vi "cDAQ_VI_Leo_Simplified.vi"() -> ()   [LabVIEW 2022 SP3]
uses:
  <vilib>/addons/control/pid/autopid.llb/PID autotuning parameters.ctl
  <vilib>/Analysis/baseanly.llb/Mean (DBL).vi
  <vilib>/DAQmx/read.llb/DAQmx Read (Analog 1D Wfm NChan NSamp).vi
  <vilib>/DAQmx/configure/timing.llb/DAQmx Timing (Sample Clock).vi
  STOP_GLOBAL.vi
  <vilib>/addons/control/pid/pid.llb/PID Lead-Lag (DBL).vi
  <vilib>/addons/control/pid/pid.llb/PID Gain Schedule (DBL).vi
  <vilib>/addons/control/pid/autopid.llb/PID Online Autotuning (Step Closed Loop).vi
  <vilib>/addons/control/pid/pid.llb/PID Advanced (DBL).vi
  <vilib>/addons/control/pid/pid.llb/PID (DBL).vi
  <vilib>/DAQmx/miscellaneous.llb/DAQmx Fill In Error Info.vi
  <vilib>/Analysis/NI_AALBase.lvlib
  <vilib>/addons/control/pid/NI_PID_pid.lvlib
  <vilib>/ptbypt/NI_PtbyPt.lvlib
  <vilib>/addons/control/pid/NI_PID_autopid.lvlib
  <resource>/objmgr/daqmx.rc
panel:
  out "Runtime Passed?":bool
  out "Stop":bool
  out "Elapsed Time (s)":dbl
  out "2nd Loop Time":dbl
  out "Numeric":i32
  out "Array":dbl[](array[numeric])
  in  "RunTime":dbl
  out "Entire Runtime":dbl
  out "Actual Clock Rate":dbl
  in  "MV:":dbl(slide)=30.8641975308642 scale=0.0..5.067 scale format="%.1f"
  in  "autotuning parameters":T1={"type of controller"=0, "relay cycles"=3, "relay amplitude"=1.0, "control specifications"=2, "PV noise level"=0.1} {"PV noise level" format="%.2f"; "control specifications" items=["normal", "fast", "slow"]; "relay amplitude" format="%.2f"; "type of controller" items=["P", "PI", "PID"]}
  in  "PID gain schedule":T2(array[cluster])=[{"PID gains"={"Kc"=7.0, "Ti"=0.001, "Td"=0.0}, "max value"=0.0}] {"max value" format="%.2f"; "PID gains"."Td" format="%#.3g"; "PID gains"."Ti" format="%#.3g"; "PID gains"."Kc" format="%#.3g"}
  out "error out 4":errorcluster
  out "Setpoint profile":dbl
  out "Voltage Output":dynamicdata(graph)
  out "Second Pressure Transducer":cluster{dbl[], dbl[]}(graph)
  out "Second Pressure Transducer":dynamicdata(graph)
  out "Servo Voltage Output":cluster{dbl[], dbl[]}(graph)
  in  "Tab Control":T3(tab)
  in  "Channel Array":dbl[](array[numeric]) format="%_3g"
  out "error out 5":errorcluster
  in  "stop":bool
  in  "Array 2":dbl[](array[slide]) scale=0.0..1.0
  out "Waveform Chart":cluster{"SP":dbl, dbl}(graph)
  out "Output":dbl(slide) scale=1.0..5.067
  out "Process Variable vs Setpoint":cluster{dbl[], dbl[]}[](graph)
  out "error out":errorcluster
  in  "Error":dbl
  in  "Scaling Factor":dbl
  in  "x0":dbl
  out "element":dbl
  out "MVT Process variable":dbl
  out "MVT Setpoint":dbl
  out "Gain Index":i32
  in  "SP":dbl format="%.2f"
  out "PID gains out":T4={"proportional gain (Kc)"=1.0, "integral time (Ti, min)"=0.01, "derivative time (Td, min)"=0.0} {"derivative time (Td, min)" format="%.3f"; "integral time (Ti, min)" format="%.3f"; "proportional gain (Kc)" format="%.3f"}
  in  "Insert Gain":bool
  out "output":dbl format="%.2f"
  in  "Autotune":bool
  in  "Reinitialize":bool
  in  "Automatic":bool=TRUE
  in  "Replace Gain":bool
  in  "alpha":dbl=nan format="%.2f"
  out "tuned PID gains":T4={"proportional gain (Kc)"=1.0, "integral time (Ti, min)"=0.01, "derivative time (Td, min)"=0.0} {"derivative time (Td, min)" format="%.3f"; "integral time (Ti, min)" format="%.3f"; "proportional gain (Kc)" format="%.3f"}
  out "Steps on Servo":dbl[](array[numeric])
  out "Elapsed Time (s) 2":dbl caption="Elapsed Time (s)"
  out "HAS 3 SECONDS PASSED?":bool
  in  "PRESS TO START":bool
  out "All Channel Graph":cluster{dbl[], dbl[]}[](graph)
  out "Thrust":cluster{dbl[], dbl[]}(graph)
  out "Chamber Pressure":cluster{dbl[], dbl[]}(graph)
  out "Supply Pressure":cluster{dbl[], dbl[]}(graph)
  out "MassFlow":cluster{dbl[], dbl[]}(graph)
  out "Temperature":cluster{dbl[], dbl[]}(graph)
  out "error out 3":errorcluster caption="error out"
  out "error out 2":errorcluster
  in  "rate":dbl=1000.0 format="%0.2f"
  in  "number of samples":i32=100
  in  "File Format":string
  in  "File Name Out":string
  in  "Data Collection Folder":path
  out "Temperature":dynamicdata(graph)
  out "Numeric 2":i32
  out "Thrust lb":dynamicdata(graph)
  in  "Types of Testing":enum32{"Test Firing", "Cold Flow Rig"}(tab)
  out "Saving Data":bool
  out "Filename Out":path
  in  "Collect Data?":bool=TRUE caption="Enable"
  in  "Collect Data? 2":bool=TRUE caption="Enable"
  out "Saving Data":bool
  out "Filename Out":path
  out "Supply Pressure PSI":dynamicdata(graph)
  out "Mass Flow L/min":dynamicdata(graph)
  out "Chamber Pressure":dynamicdata(graph)
  # "Control Loop"
  # "DATA LOGGING INFORMATION"
  # "ANALOG VOLTAGE OUTPUT"
  # "RESULTS"
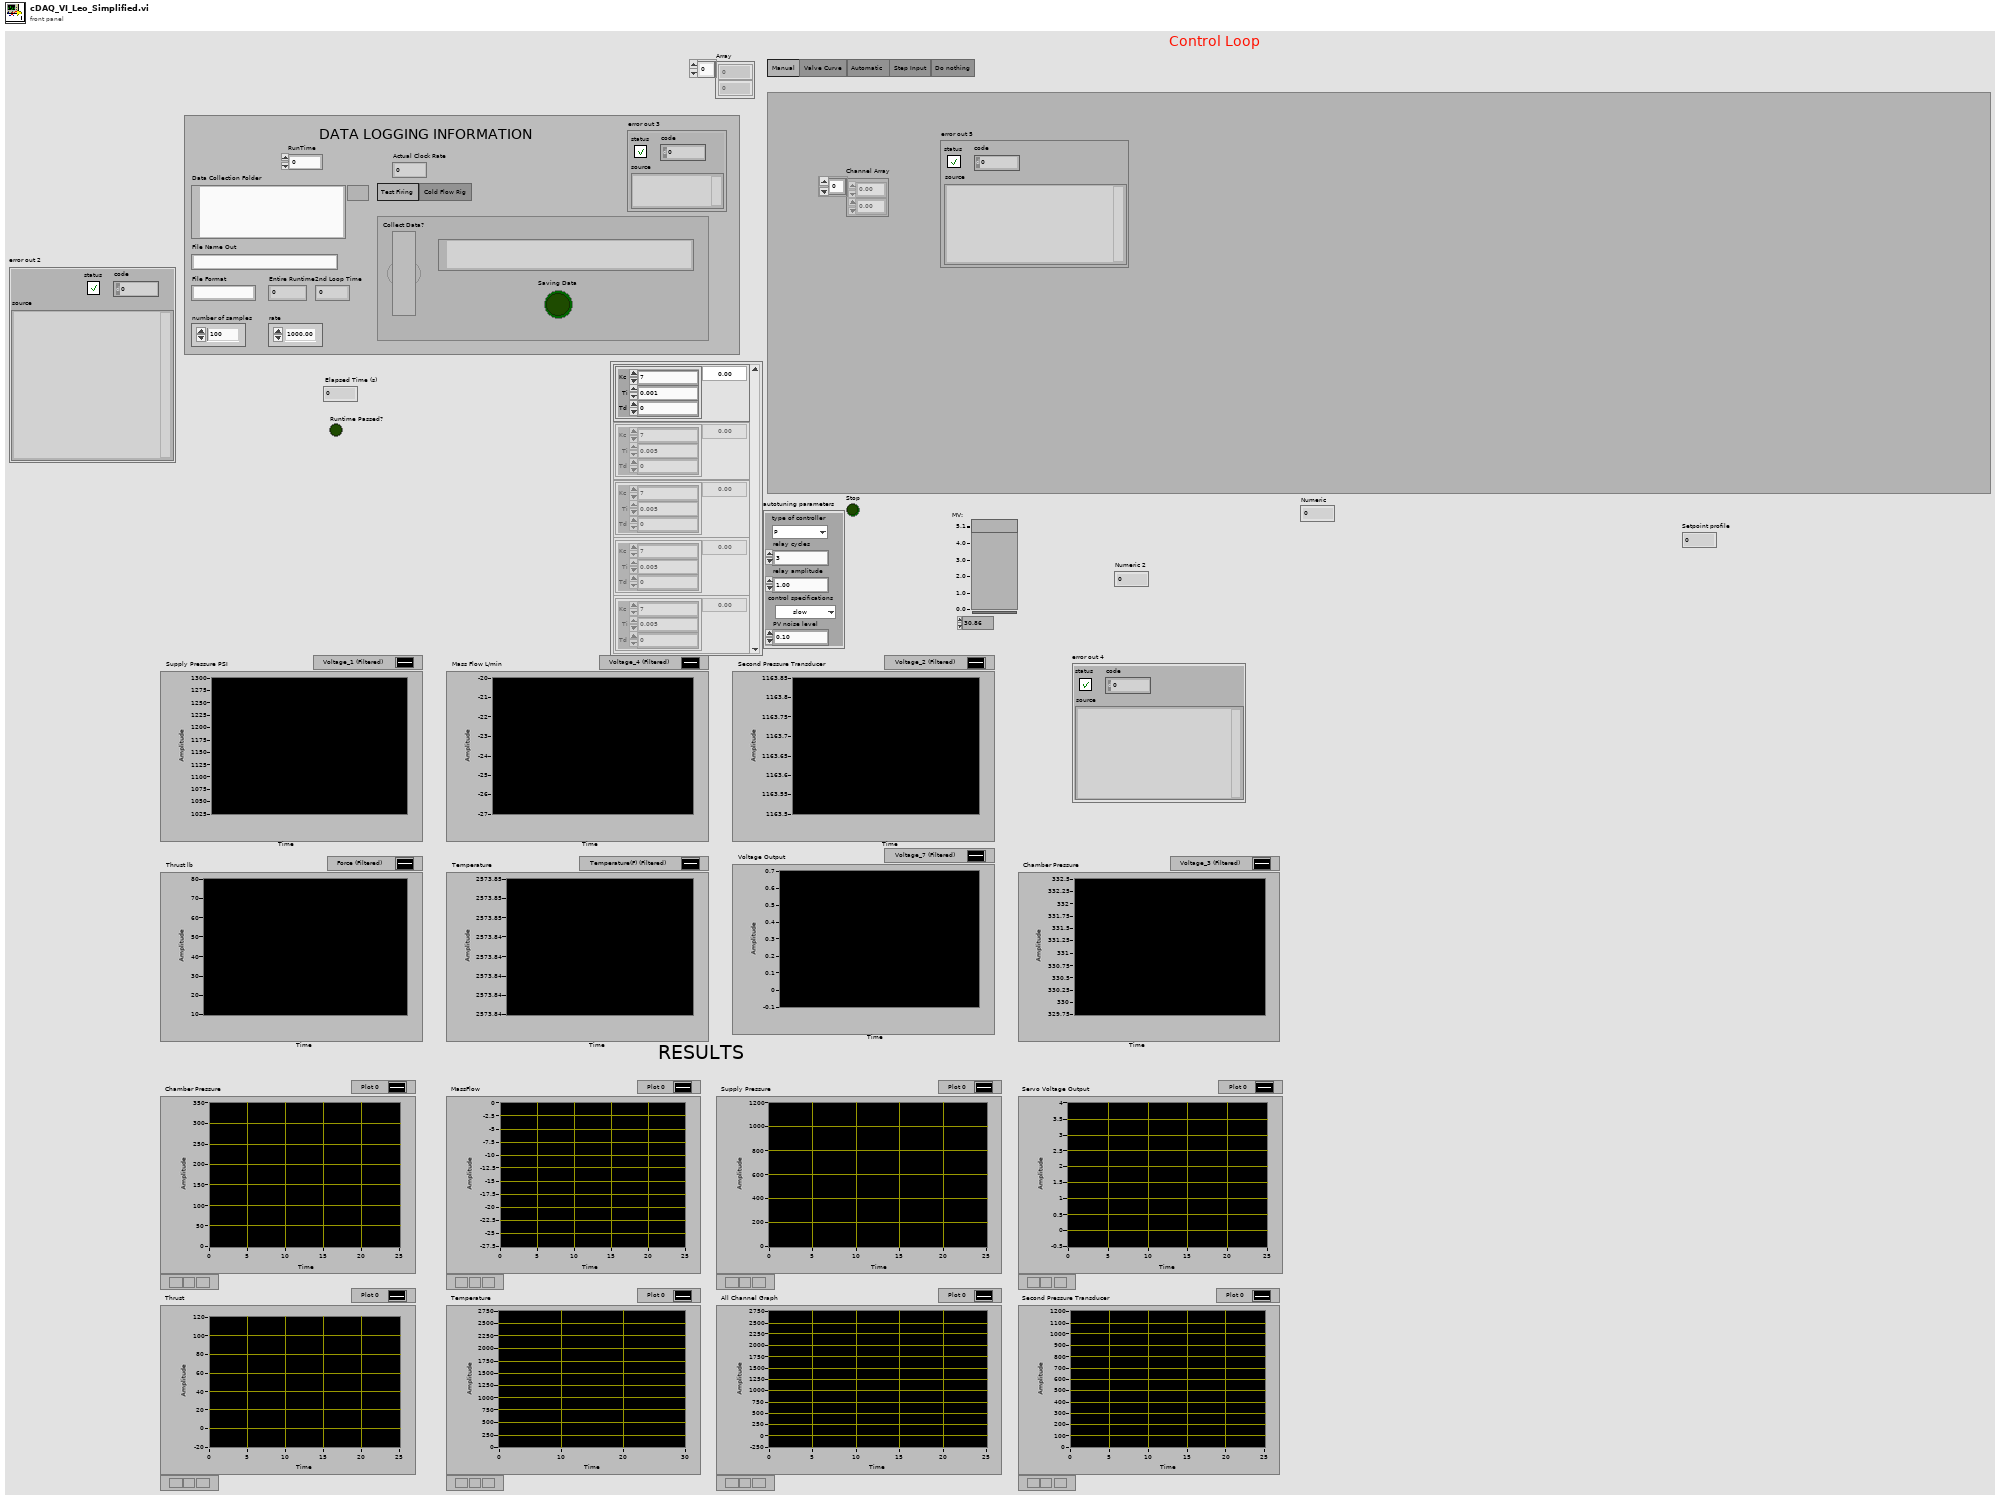
[diagram p1: front panel]
types:
  T1 = typedef "PID autotuning parameters.ctl" = cluster{"type of controller":u16, "relay cycles":i32, "relay amplitude":dbl, "control specifications":u16, "PV noise level":dbl}
  T2 = cluster{"PID gains":cluster{"Kc":dbl, "Ti":dbl, "Td":dbl}, "max value":dbl}[]
  T3 = enum32{"Manual", "Valve Curve", "Automatic", "Step Input", "Do nothing"}
  T4 = cluster{"proportional gain (Kc)":dbl, "integral time (Ti, min)":dbl, "derivative time (Td, min)":dbl}
  T5 = cluster{"tuned PID gains":cluster{"proportional gain (Kc)":dbl, "integral time (Ti, min)":dbl, "derivative time (Td, min)":dbl}, "SP":dbl}
  T6 = cluster{"PID gains":cluster{"Kc":dbl, "Ti":dbl, "Td":dbl}, "max value":dbl}
  T7 = cluster{"tuned PID gains":cluster{"proportional gain (Kc)":dbl, "integral time (Ti, min)":dbl, "derivative time (Td, min)":dbl}, "max value":dbl}
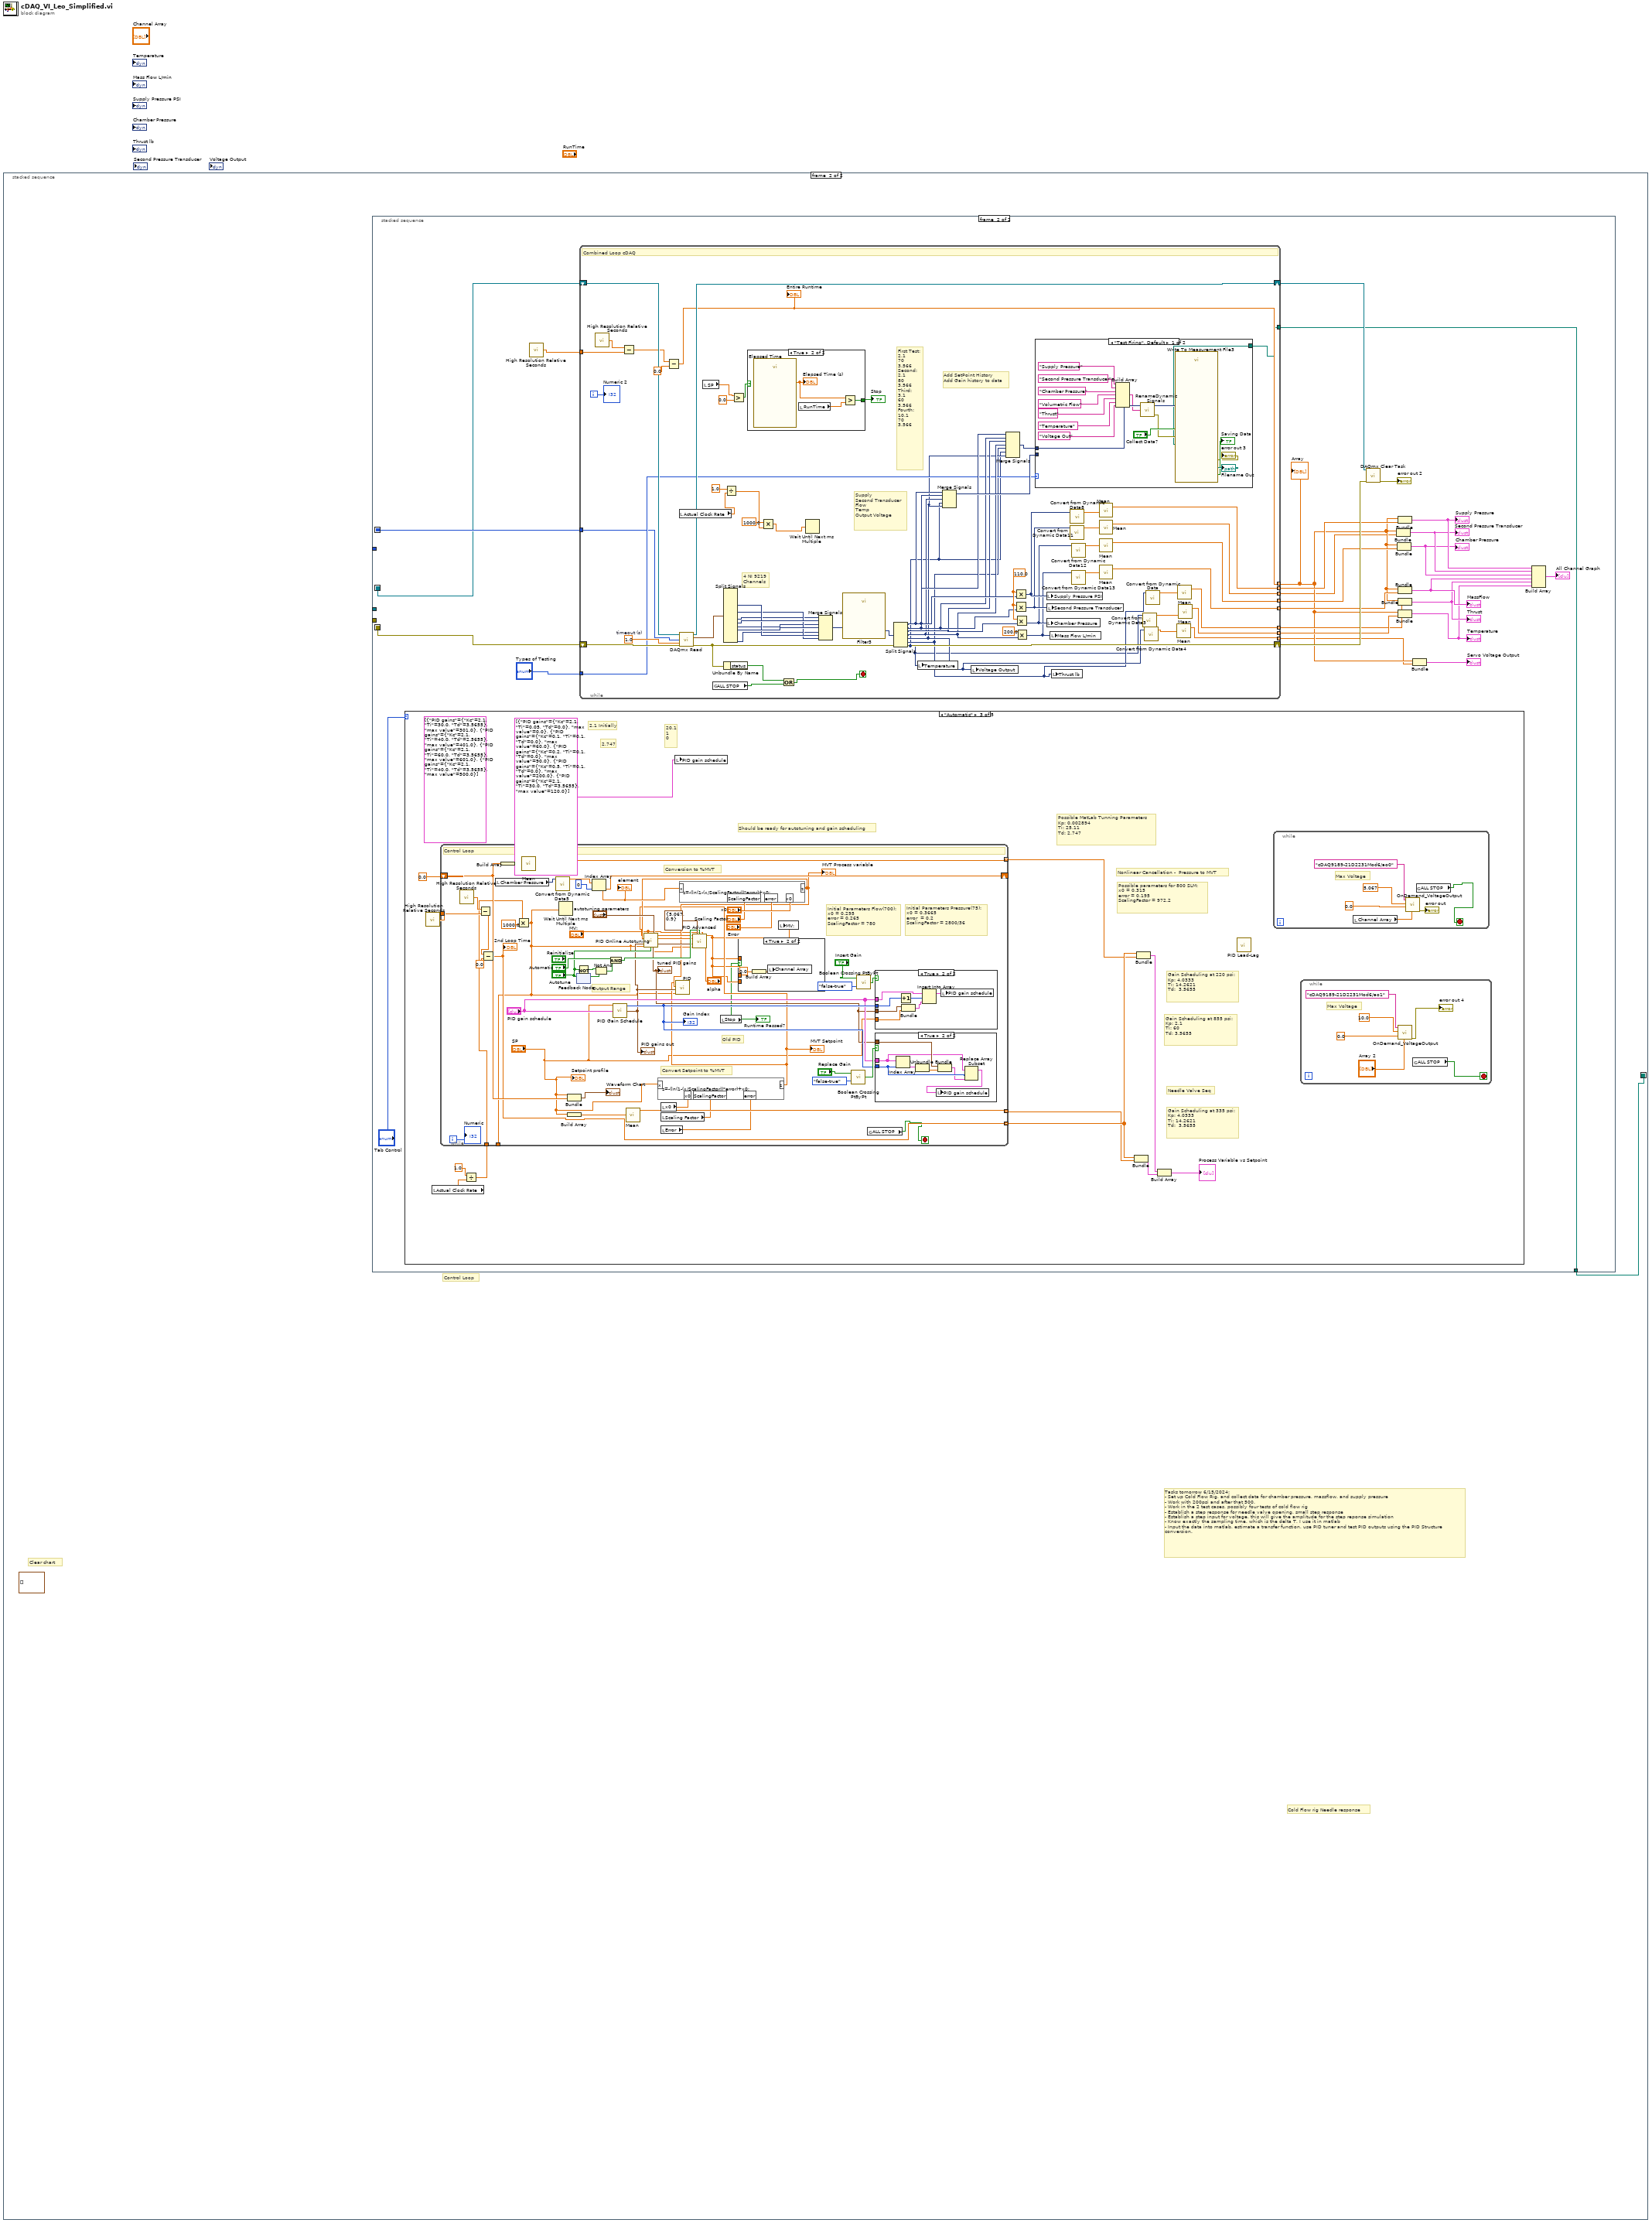
[diagram p0: block diagram]
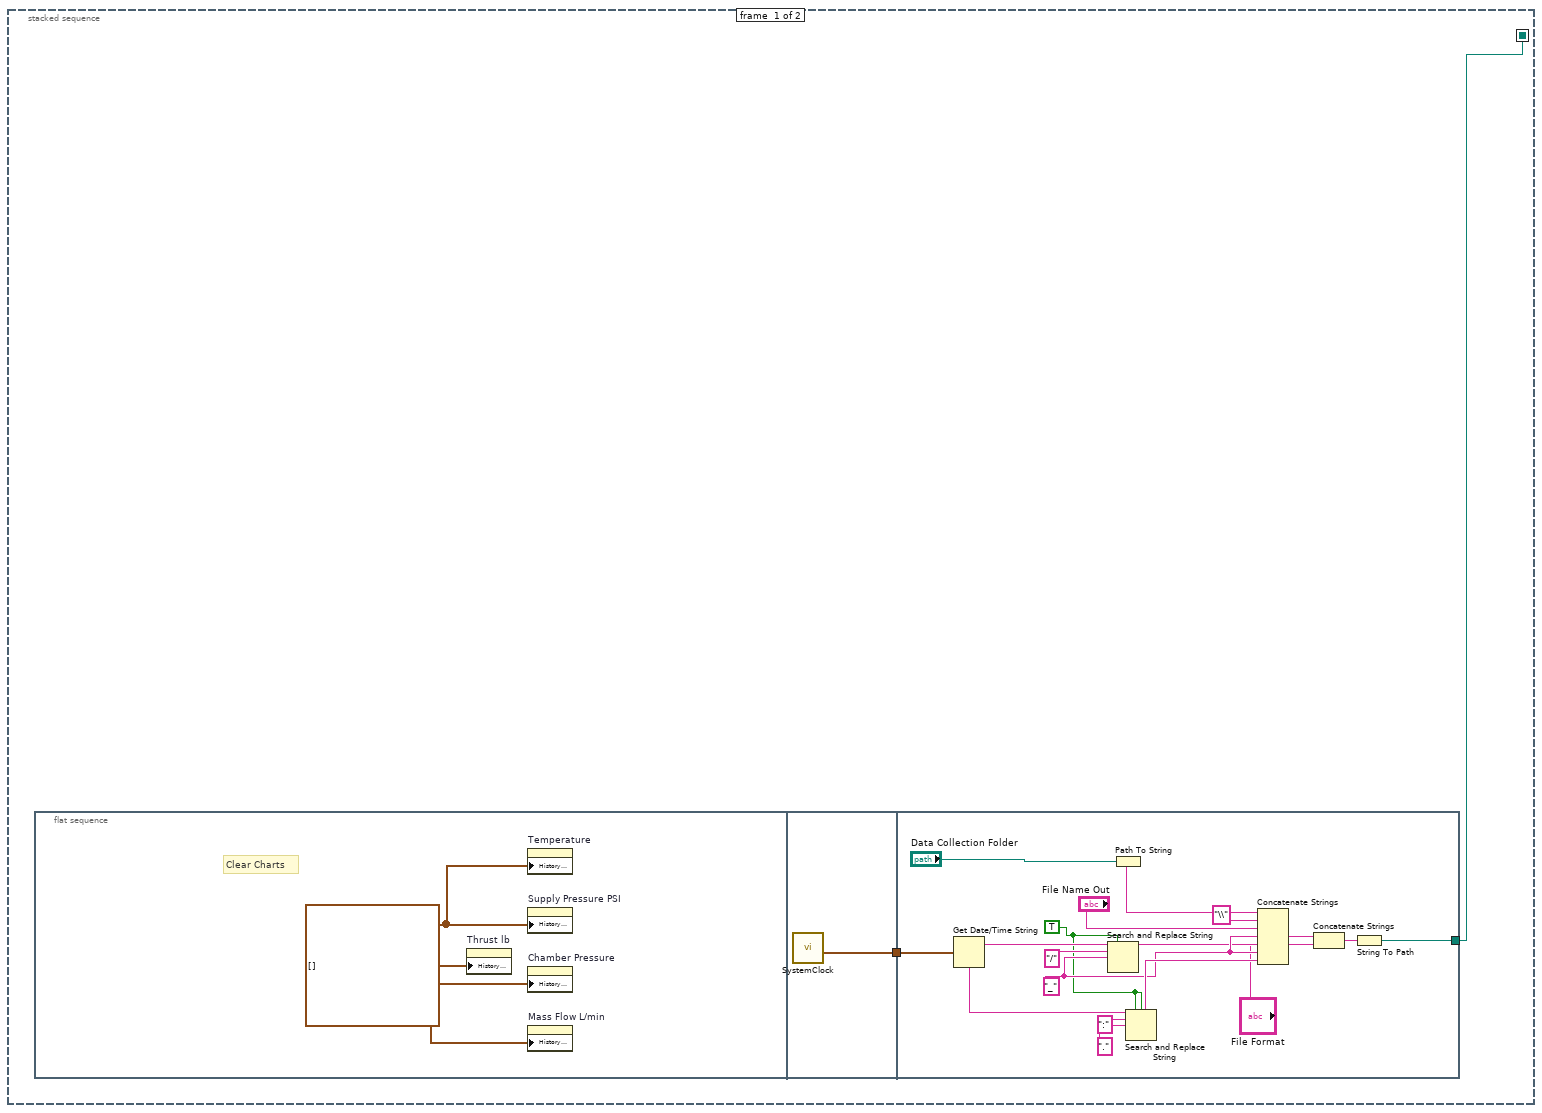
[diagram p2: hidden frame]
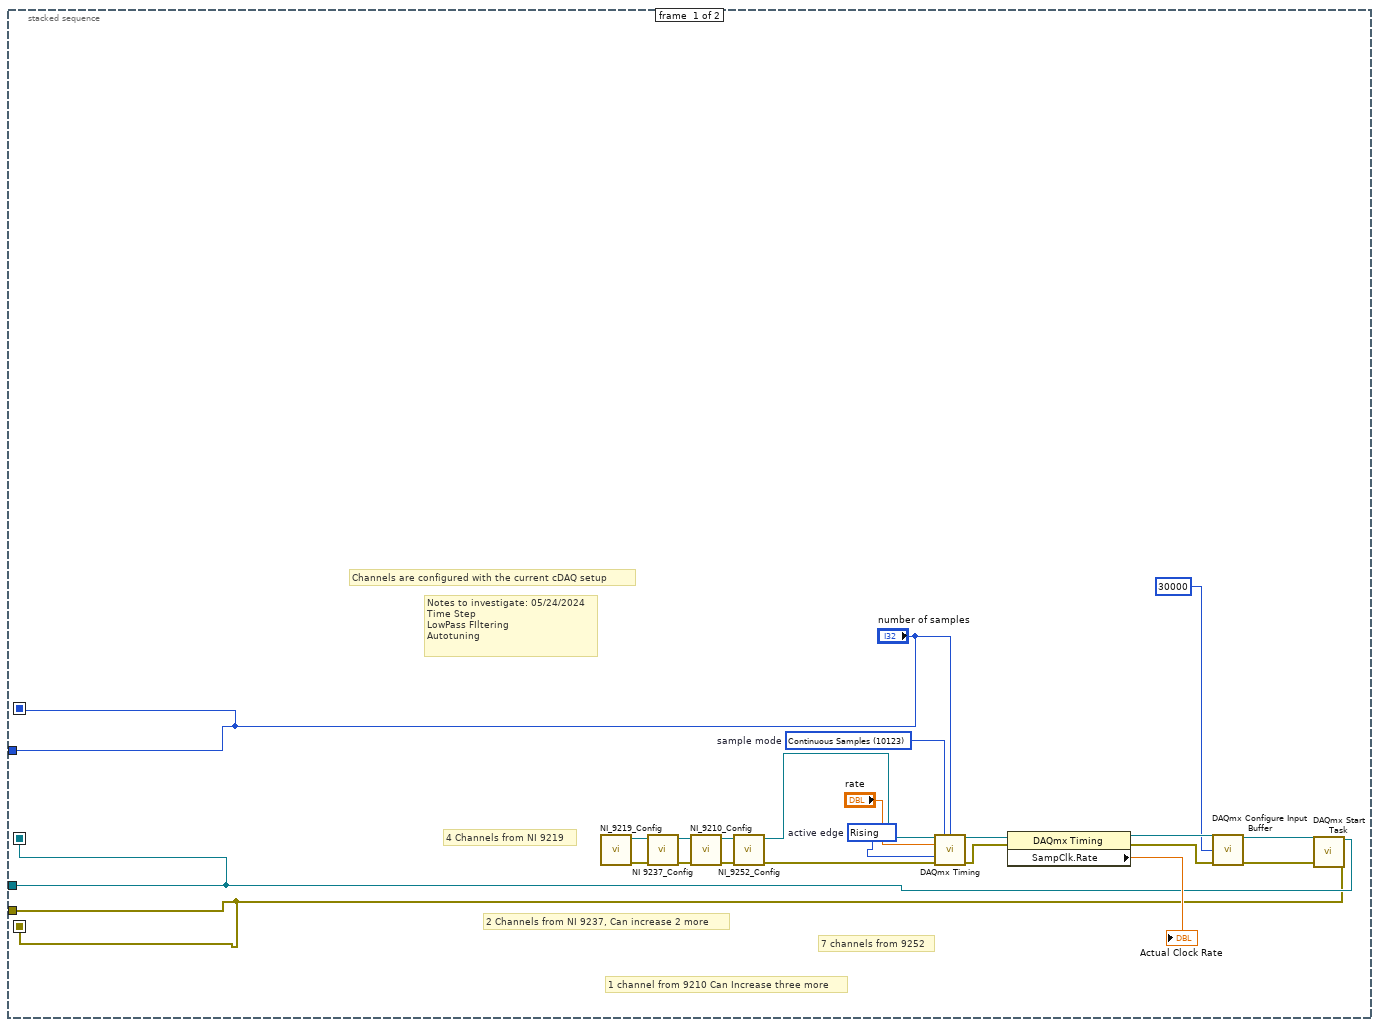
[diagram p3: hidden frame]
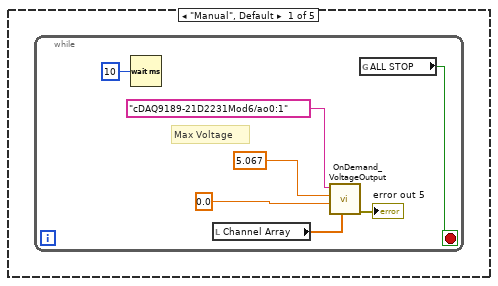
[diagram p4: hidden frame]
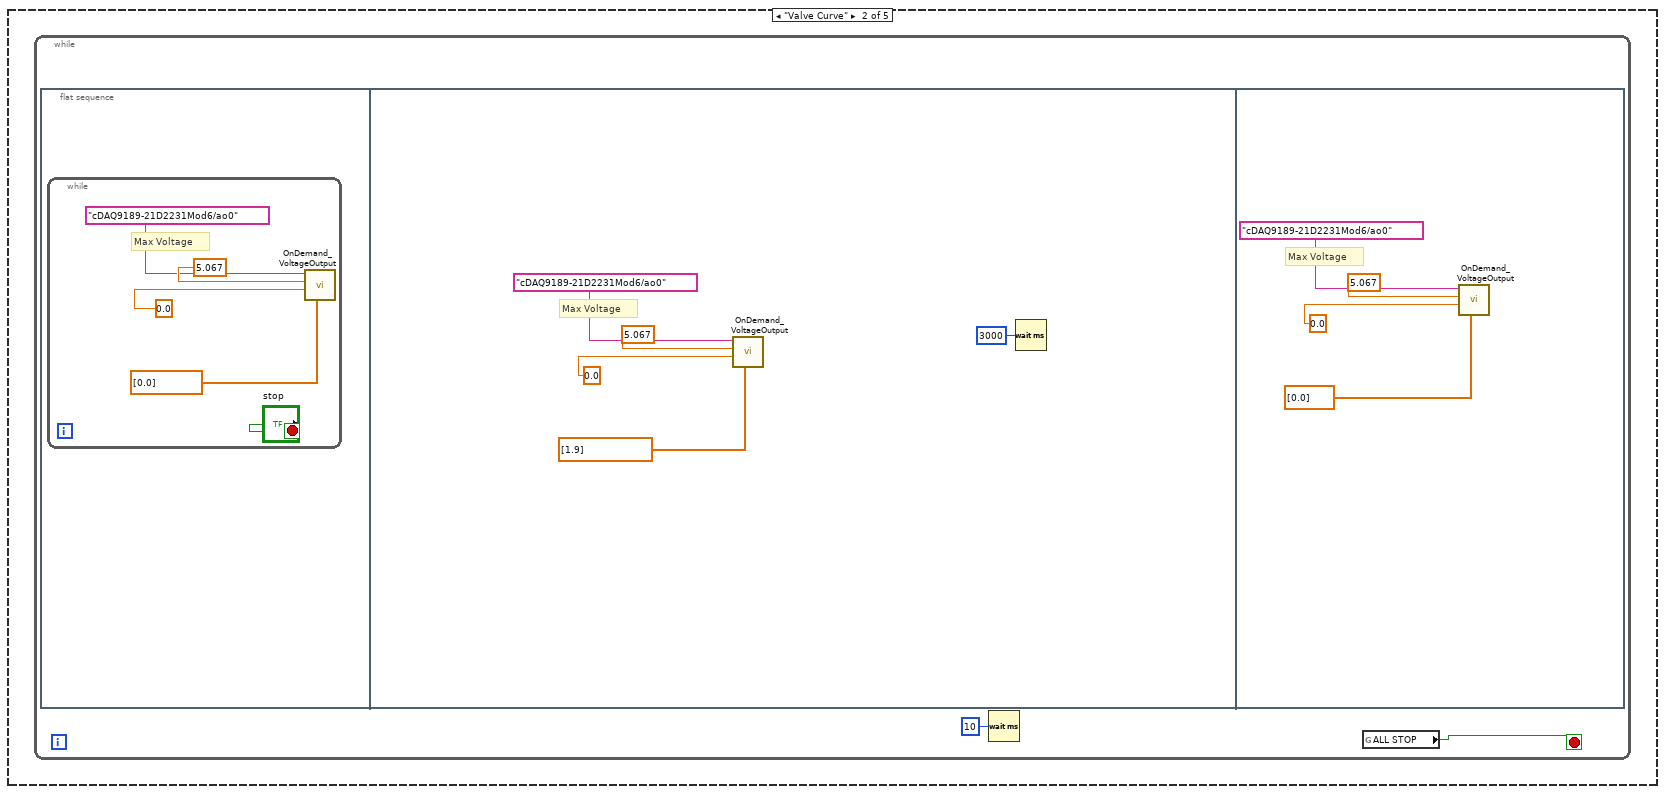
[diagram p5: hidden frame]
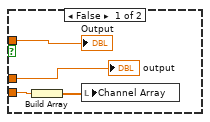
[diagram p6: hidden frame]
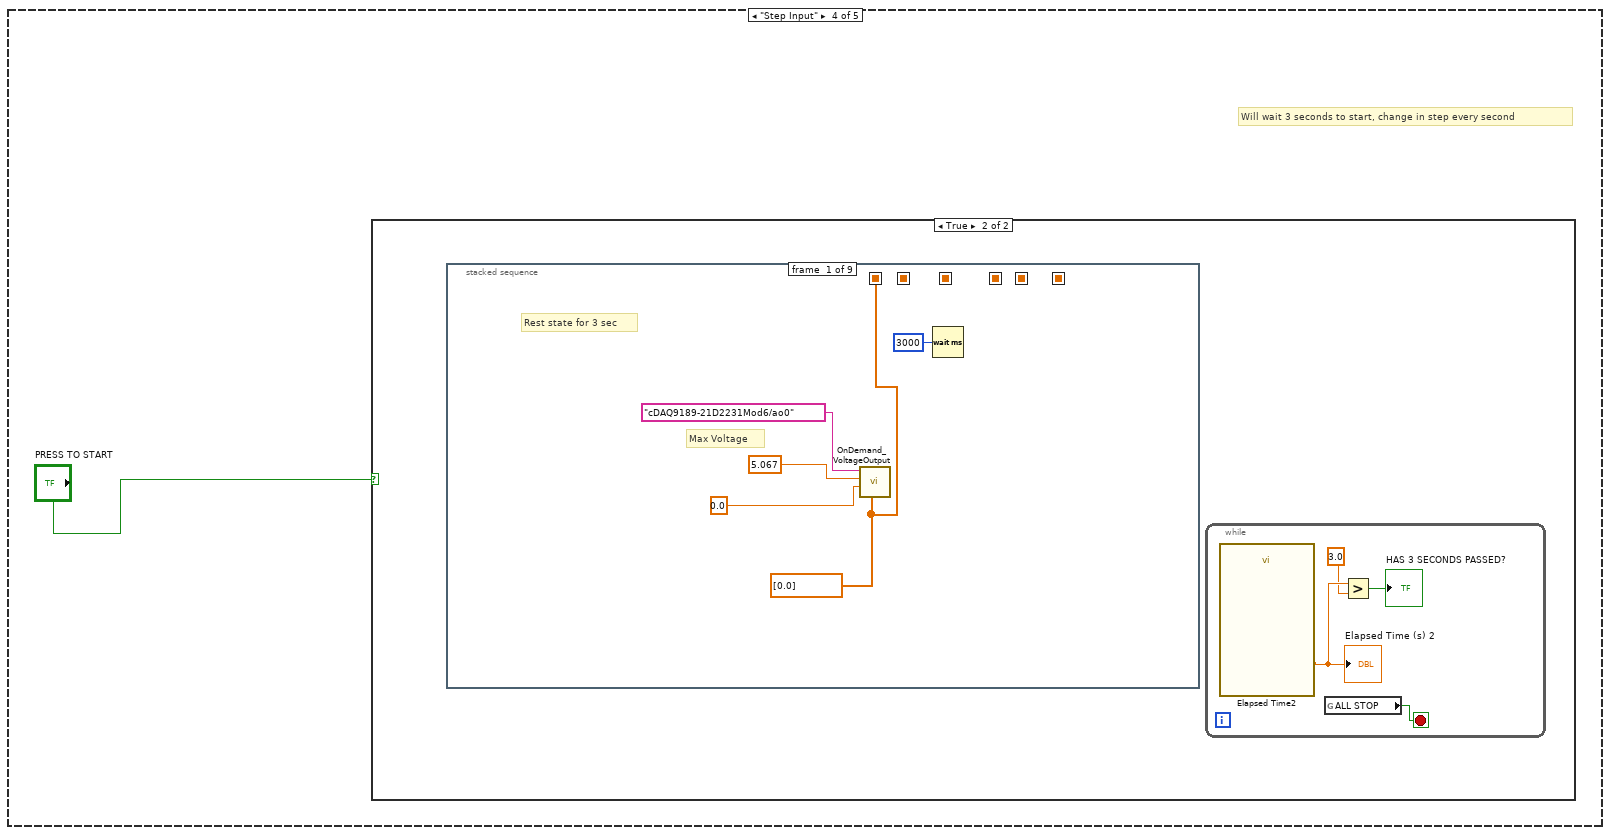
[diagram p9: hidden frame]
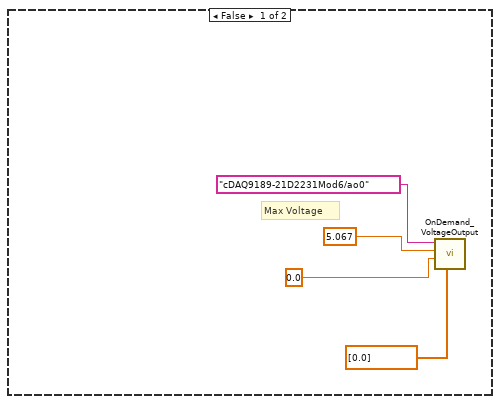
[diagram p10: hidden frame]
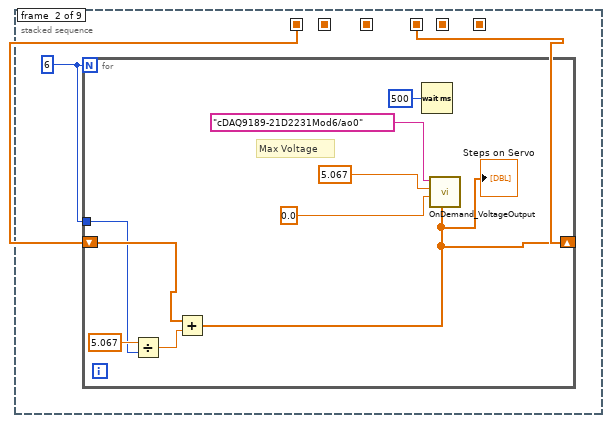
[diagram p11: hidden frame]
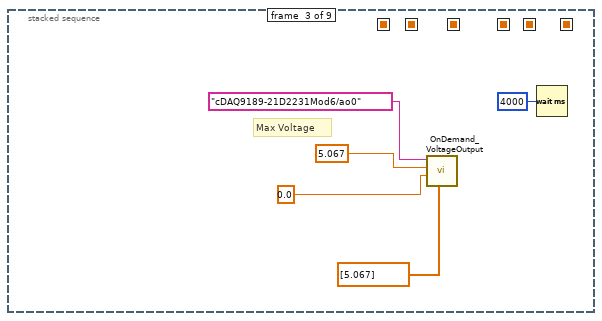
[diagram p12: hidden frame]
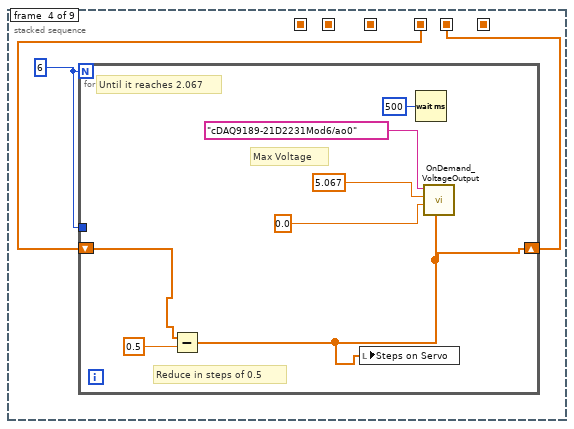
[diagram p13: hidden frame]
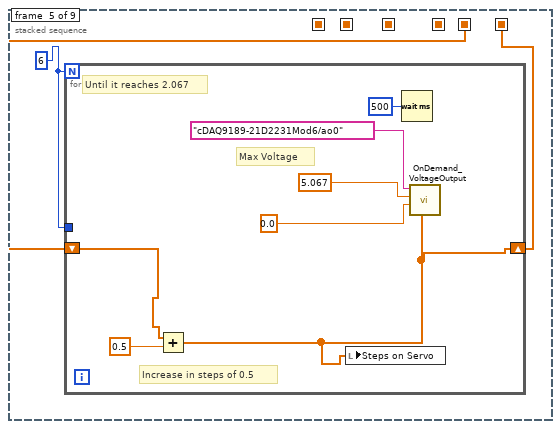
[diagram p14: hidden frame]
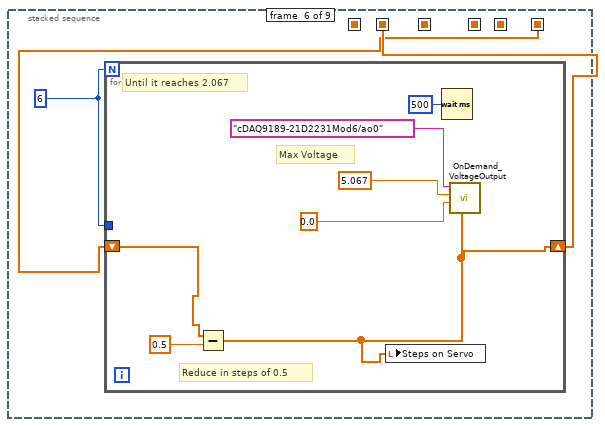
[diagram p15: hidden frame]
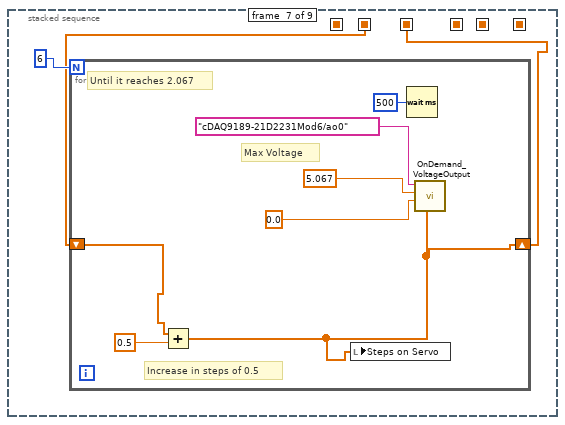
[diagram p16: hidden frame]
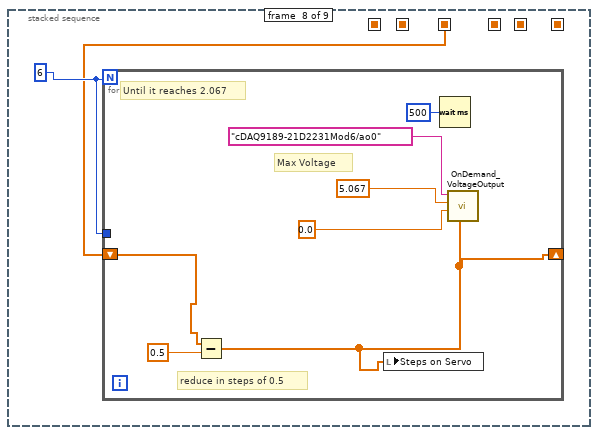
[diagram p17: hidden frame]
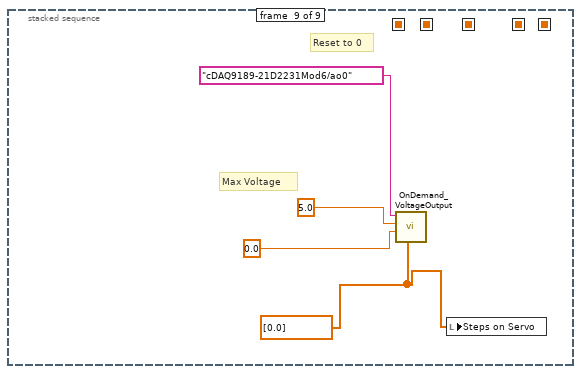
[diagram p18: hidden frame]
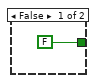
[diagram p20: hidden frame]
diagram:
  n1 = stacked-sequence {
    seq-local: [w1 _] -> [_ w23]
    frame #0 {
      n2 = flat-sequence {
        tunnel: [w4] -> w2
        tunnel: w2 -> [w11]
        tunnel: [w10] -> w1
        frame #0 {
          w3 = waveform(dbl)[] []
          # "Clear Charts"
          n3 = property on="Thrust lb" class="WFChart (strict)"("History Data"=w3) -> ()  [unwired: 2 in, 2 out]
          n4 = property on="Temperature" class="WFChart (strict)"("History Data"=w3) -> ()  [unwired: 2 in, 2 out]
          n5 = property on="Supply Pressure PSI" class="WFChart (strict)"("History Data"=w3) -> ()  [unwired: 2 in, 2 out]
          n6 = property on="Chamber Pressure" class="WFChart (strict)"("History Data"=w3) -> ()  [unwired: 2 in, 2 out]
          n7 = property on="Mass Flow L/min" class="WFChart (strict)"("History Data"=w3) -> ()  [unwired: 2 in, 2 out]
        }
        frame #1 {
          n8 = call "SystemClock.vi"() -> ("LabVIEW Time Stamp"=w4:timestamp)  [unwired: 9 in, 2 out]
        }
        frame #2 {
          w6 = TRUE ("replace all? (F)")
          w19 = "_" ("string")
          n9 = Get Date/Time String(seconds (now)=w11) -> (date string=w13:string, time string=w16:string)  [unwired: 2 in]
          n10 = Search and Replace String(replace all?=w6, input string=w13, search string="/", replace string=w19) -> (result string=w15:string)  [unwired: 4 in, 3 out]
          n11 = Path To String(path="Data Collection Folder") -> (string=w8:string)
          n12 = Search and Replace String(replace all?=w6, case sensitive?=w6, input string=w16, search string=":", replace string="." ("replace string (\"\")")) -> (result string=w20:string)  [unwired: 3 in, 3 out]
          n13 = Concatenate Strings(w8, "\\" ("string"), "File Name Out", w19, w15, w19, w20) -> (w21:string)
          n14 = Concatenate Strings(w21, "File Format") -> (w22:string)
          n15 = String To Path(string=w22) -> (path=w10:path)
        }
      }
    }
    frame #1 {
      (unwired) cluster{"setpoint":dbl, dbl}[] [] ("History Data")
      # "Cold Flow rig Needle response"
      # "Tasks tomorrow 6/15/2024:\n- Set up Cold Flow Rig, and collect data for chamber pressure, massflow, and supply pressure\n- Work with 200psi and after that 500.\n- Work in the 2 test cases, possibly four tests of cold flow rig\n- Establish a step response for needle valve opening, small step response\n- Establish a step input for voltage, this will give the amplitude for the step reponse simulation\n- Know exactly the sampling time, which is the delta T, I use it in matlab\n- Input the data into matlab, estimate a transfer function, use PID tuner and test PID outputs using the PID Structure\nconversion."
      # "Control Loop"
      # "Clear chart"
      n16 = stacked-sequence {
        seq-local: ["number of samples" _] -> [_ w50]
        seq-local: [w25 _] -> [_ w49]
        seq-local: [w24 _] -> [_ w48]
        tunnel: w23 -> [_ w46]
        tunnel: [w25 _] -> _
        tunnel: [w24 _] -> _
        tunnel: ["number of samples" _] -> _
        frame #0 {
          w28 = 10123 items=["Finite Samples"=10178, "Continuous Samples"=10123, "Hardware Timed Single Point"=12522]  # sample mode
          w27 = 10280 items=["Rising"=10280, "Falling"=10171]  # active edge
          # "Notes to investigate: 05/24/2024\nTime Step\nLowPass FIltering\nAutotuning"
          # "Channels are configured with the current cDAQ setup"
          # "7 channels from 9252"
          # "1 channel from 9210 Can Increase three more"
          # "2 Channels from NI 9237, Can increase 2 more"
          # "4 Channels from NI 9219"
          n17 = call "NI_9219_Config.vi"() -> ("error out"=w38:errorcluster, "task out"=w30:refnum<k21>)  [unwired: 10 in]
          n18 = call "NI 9237_Config.vi"("error in"=w38, "task in"=w30) -> ("error out"=w32:errorcluster, "task out"=w31:refnum<k21>)  [unwired: 8 in]
          n19 = call "NI_9210_Config.vi"("error in"=w32, "task in"=w31) -> ("error out"=w34:errorcluster, "task out"=w33:refnum<k21>)  [unwired: 8 in]
          n20 = call "NI_9252_Config.vi"("error in"=w34, "task in"=w33) -> ("error out"=w36:errorcluster, "task out"=w35:refnum<k21>)  [unwired: 8 in]
          n21 = call-poly <vilib>:"DAQmx Timing.vi"("task/channels in"=w35, "sample mode"=w28, "samples per channel"="number of samples", "rate"="rate", "active edge"=w27, "error in"=w36) -> ("task out"=w39:refnum<k21>, "error out"=w40:errorcluster)  [unwired: 8 in]
          n22 = property class="DAQmx Timing"(reference=w39, error in=w40) -> (reference out=w41:refnum<k21>, error out=w42:errorcluster, "SampClk.Rate"=→"Actual Clock Rate":dbl)
          n23 = call <vilib>:"DAQmx Configure Input Buffer.vi"("task/channels in"=w41, "buffer size (in samples per channel)"=u32 30000, "error in"=w42) -> ("task out"=w44:refnum<k21>, "error out"=w43:errorcluster)  [unwired: 11 in]
          n24 = call <vilib>:"DAQmx Start Task.vi"("task/channels in"=w44, "error in"=w43) -> ("task out"=w25:refnum<k21>, "error out"=w24:errorcluster)  [unwired: 12 in]
        }
        frame #1 {
          n25 = case shown="\"Automatic\"" "Tab Control" {
            frame "Manual", Default {
              n26 = while {
                stop <- w78 stop-if-true
                # "Max Voltage"
                n27 = Wait (ms)(milliseconds to wait=u32 10) -> ()  [unwired: 1 out]
                n28 = local read "Channel Array"() -> (w74:dbl[])
                n29 = call "OnDemand_VoltageOutput.vi"("Channel Array"=w74, "minimum voltage"=0.0, "maximum voltage"=5.067, "physical channels"="cDAQ9189-21D2231Mod6/ao0:1") -> ("error out"=→"error out 5":errorcluster)  [unwired: 7 in]
                n30 = global read "STOP_GLOBAL.vi" "ALL STOP"() -> (w78:bool)
              }
            }
            frame "Valve Curve" {
              n31 = while {
                stop <- w79 stop-if-true
                n32 = flat-sequence {
                  frame #0 {
                    n33 = while {
                      stop <- "stop" stop-if-true
                      # "Max Voltage"
                      n34 = call "OnDemand_VoltageOutput.vi"("Channel Array"=dbl[] [0.0], "minimum voltage"=0.0, "maximum voltage"=5.067, "physical channels"="cDAQ9189-21D2231Mod6/ao0") -> ()  [unwired: 7 in, 1 out]
                    }
                  }
                  frame #1 {
                    # "Max Voltage"
                    n35 = call "OnDemand_VoltageOutput.vi"("Channel Array"=dbl[] [1.9], "minimum voltage"=0.0, "maximum voltage"=5.067, "physical channels"="cDAQ9189-21D2231Mod6/ao0") -> ()  [unwired: 7 in, 1 out]
                    n36 = Wait (ms)(milliseconds to wait=u32 3000) -> ()  [unwired: 1 out]
                  }
                  frame #2 {
                    # "Max Voltage"
                    n37 = call "OnDemand_VoltageOutput.vi"("Channel Array"=dbl[] [0.0], "minimum voltage"=0.0, "maximum voltage"=5.067, "physical channels"="cDAQ9189-21D2231Mod6/ao0") -> ()  [unwired: 7 in, 1 out]
                  }
                }
                n38 = Wait (ms)(milliseconds to wait=u32 10) -> ()  [unwired: 1 out]
                n39 = global read "STOP_GLOBAL.vi" "ALL STOP"() -> (w79:bool)
              }
            }
            frame "Automatic" {
              (unwired) T2 [{"PID gains"={"Kc"=2.1, "Ti"=30.0, "Td"=3.5655}, "max value"=301.0}, {"PID gains"={"Kc"=2.1, "Ti"=40.0, "Td"=2.5655}, "max value"=401.0}, {"PID gains"={"Kc"=2.1, "Ti"=60.0, "Td"=3.5655}, "max value"=601.0}, {"PID gains"={"Kc"=2.1, "Ti"=40.0, "Td"=3.5655}, "max value"=500.0}] ("PID gain schedule 2")
              # "2.1 Initially"
              # "20.1\n1\n0"
              # "2.747"
              # "Should be ready for autotuning and gain scheduling"
              # "Possible parameters for 800 SLM:\nx0 = 0.315\nerror = 0.195\nScalingFactor = 972.2"
              # "Nonlinear Cancellation -  Pressure to MVT"
              # "Possible MatLab Tunning Parameters\nKp: 0.002894\nTi: 25.11\nTd: 2.747"
              # "Gain Scheduling at 335 psi:\nKp: 4.0333\nTi: 14.2621\nTd:  3.5655"
              # "Gain Scheduling at 855 psi:\nKp: 2.1\nTi: 60\nTd: 3.5655"
              # "Gain Scheduling at 220 psi:\nKp: 4.0333\nTi: 14.2621\nTd:  3.5655"
              # "Needle Valve Seq"
              n40 = call <vilib>:"High Resolution Relative Seconds.vi"() -> ("relative seconds"=w98:dbl)
              n41 = local read "Actual Clock Rate"() -> (w97:dbl)
              n42 = Divide(x=1.0, y=w97) -> (x/y=w95:dbl)
              n43 = while {
                shift-right: [w136] -> _
                shift-left: 0.0 -> [w171]
                tunnel: [w127] -> w104 mode=indexing
                tunnel: [w170] -> w102 mode=indexing
                tunnel: [w168] -> w103 mode=indexing
                tunnel: w98 -> [w131]
                tunnel: [w126] -> _
                tunnel: w95 -> [w125]
                i -> [w132]
                stop <- w120 stop-if-true
                # "Old PID"
                # "Initial Parameters Pressure(75):\nx0 = 0.3665\nerror  = 0.2\nScalingFactor = 2800/36"
                # "Initial Parameters Flow(700):\nx0 = 0.295\nerror = 0.265\nScalingFactor = 780"
                # "Convert Setpoint to %MVT"
                # "Conversion to %MVT"
                # "Output Range"
                # "Control Loop"
                n44 = call <vilib>:"High Resolution Relative Seconds.vi"() -> ("relative seconds"=w130:dbl)
                n45 = Subtract(x=w130, y=w131) -> (x-y=w129:dbl)
                n46 = Subtract(x=w129, y=0.0) -> (x-y=w127:dbl)
                "2nd Loop Time" <- w127
                n47 = local read "Chamber Pressure"() -> (w122:dynamicdata)
                n48 = Build Array(w171) -> (w169:dbl[])
                n49 = Multiply(x=w125, y=1000.0) -> (x*y=w126:dbl)
                n50 = call-poly <vilib>:"Mean.vi"("X"=w169) -> ("mean"=w170:dbl)  [unwired: 1 out]
                n51 = call "Convert from Dynamic Data5"("Dynamic Data Type"=w122) -> ("Array"=w160:dbl[])  [unwired: 3 in]
                n52 = Wait Until Next ms Multiple(millisecond multiple=w126) -> ()  [unwired: 1 out]
                n53 = Bundle("SP"="SP", w171) -> (→"Waveform Chart":cluster{"SP":dbl, dbl})  [unwired: 1 in]
                n54 = Build Array("SP") -> (w166:dbl[])
                n55 = feedback #1() -> (w155:bool)  [unwired: 1 in]
                n56 = feedback-in #1("Autotune") -> ()
                n57 = Not(x="Autotune") -> (.not. x?=w154:bool)
                n58 = Index Array(array=w160, index=0) -> (element=w136:dbl)
                "element" <- w136
                n59 = Not And(1:w155, 2:w154) -> (0:w153:bool)
                n60 = And(x="Automatic", y=w153) -> (x .and. y?=w149:bool)
                n61 = call-poly <vilib>:"PID Gain Schedule.vi"("PID gain schedule"="PID gain schedule", "gain scheduling value"="SP") -> ("PID gains out"=w139:T4, "index out"=w141:i32)  [unwired: 2 in]
                "Gain Index" <- w141
                "PID gains out" <- w139
                n62 = call-poly <vilib>:"Mean.vi"("X"=w166) -> ("mean"=w168:dbl)  [unwired: 1 out]
                n63 = local read "x0"() -> (w165:dbl)
                n64 = local read "Scaling Factor"() -> (w156:dbl)
                n65 = local read "Error"() -> (w164:dbl)
                n66 = formula code="z=-(ln(1-(x/ScalingFactor))*error)+x0;"("x"="SP", "x0"=w165, "ScalingFactor"=w156, "error"=w164) -> ("z"=w134:dbl)
                "MVT Setpoint" <- w134
                n67 = formula code="z=-(ln(1-(x/ScalingFactor))*error)+x0;"("x"=w136, "x0"="x0", "ScalingFactor"="Scaling Factor", "error"="Error") -> ("z"=w135:dbl)
                "MVT Process variable" <- w135
                n68 = call-poly <vilib>:"PID Online Autotuning.vi"("setpoint"=w134, "manipulated variable"="MV:", "autotuning parameters"="autotuning parameters", "process variable"=w135, "PID gains in"=w139, "dt (s)"=w126, "autotune? (F)"="Autotune") -> ("setpoint out"=w148:dbl, "process variable out"=w147:dbl, "PID gains out"=w146:T4, "tuned PID gains"=w137:T4)  [unwired: 4 in, 1 out]
                "tuned PID gains" <- w137
                n69 = call-poly <vilib>:"PID.vi"("dt (s)"=w126, "PID gains"=w139, "process variable"=w135, "setpoint"=w134) -> ()  [unwired: 6 in, 2 out]
                n70 = call-poly <vilib>:"PID Advanced.vi"("setpoint"=w148, "output range"=cluster{"output high":dbl, "output low":dbl} {"output high"=5.067, "output low"=0.9}, "auto? (T)"=w149, "manual control"="MV:", "process variable"=w147, "alpha"="alpha", "PID gains"=w146, "dt (s)"=w126) -> ("output"=w123:dbl)  [unwired: 6 in, 1 out]
                n71 = local read "Stop"() -> (w119:bool)
                "Runtime Passed?" <- w119
                n72 = case shown="True" w119 {
                  tunnel: w123 -> [w176 _]
                  tunnel: w123 -> [w175 _]
                  tunnel: w123 -> [w173 _]
                  frame False {
                    n73 = Build Array(w173) -> (w174:dbl[])
                    n74 = local write "Channel Array"(w174) -> ()
                    "Output" <- w176
                    "output" <- w175
                  }
                  frame True {
                    n75 = Build Array(0.0 ("element")) -> (w178:dbl[])
                    n76 = local write "Channel Array"(w178) -> ()
                  }
                }
                n77 = local write "MV:"(w123) -> ()
                n78 = call <vilib>:"Boolean Crossing PtByPt.vi"("direction"=enum16{"either", "false-true", "true-false"}."false-true", "input"="Replace Gain") -> ("crossing"=w142:bool)  [unwired: 1 in]
                n79 = call <vilib>:"Boolean Crossing PtByPt.vi"("direction"=enum16{"either", "false-true", "true-false"}."false-true", "input"="Insert Gain") -> ("crossing"=w158:bool)  [unwired: 1 in]
                n80 = global read "STOP_GLOBAL.vi" "ALL STOP"() -> (w120:bool)
                n81 = case shown="True" w158 {
                  tunnel: w141 -> [_ w192]
                  tunnel: "PID gain schedule" -> [_ w190]
                  tunnel: "SP" -> [_ w189]
                  tunnel: w137 -> [_ w187]
                  frame False {
                  }
                  frame True {
                    n82 = Increment(x=w192) -> (x+1=w191:i32)
                    n83 = Bundle("tuned PID gains"=w187, "SP"=w189) -> (w186:T5)  [unwired: 1 in]
                    n84 = Insert Into Array(array=w190, index=w191, new element=w186) -> (w188:T2)
                    n85 = local write "PID gain schedule"(w188) -> ()
                  }
                }
                n86 = case shown="True" w142 {
                  tunnel: w141 -> [_ w182]
                  tunnel: "PID gain schedule" -> [_ w180]
                  tunnel: w137 -> [_ w183]
                  frame False {
                  }
                  frame True {
                    n87 = Index Array(array=w180, index=w182) -> (element=w185:T6)
                    n88 = Unbundle(w185) -> ("max value"=w184:dbl)  [unwired: 1 out]
                    n89 = Bundle("tuned PID gains"=w183, "max value"=w184) -> (w181:T7)  [unwired: 1 in]
                    n90 = Replace Array Subset(array=w180, new element=w181, index=w182) -> (w179:T2)
                    n91 = local write "PID gain schedule"(w179) -> ()
                  }
                }
                "Setpoint profile" <- "SP"
                "Numeric" <- w132
              }
              n92 = local write "PID gain schedule"(T2 [{"PID gains"={"Kc"=2.1, "Ti"=0.05, "Td"=0.0}, "max value"=0.0}, {"PID gains"={"Kc"=0.1, "Ti"=0.1, "Td"=0.0}, "max value"=60.0}, {"PID gains"={"Kc"=0.2, "Ti"=0.1, "Td"=0.0}, "max value"=90.0}, {"PID gains"={"Kc"=0.5, "Ti"=0.1, "Td"=0.0}, "max value"=200.0}, {"PID gains"={"Kc"=2.1, "Ti"=30.0, "Td"=3.5655}, "max value"=120.0}] ("PID gain schedule 2")) -> ()
              n93 = Bundle(w104, w103) -> (w105:cluster{dbl[], dbl[]})  [unwired: 1 in]
              n94 = Bundle(w104, w102) -> (w100:cluster{dbl[], dbl[]})  [unwired: 1 in]
              n95 = Build Array(w100, w105) -> (→"Process Variable vs Setpoint":cluster{dbl[], dbl[]}[])
              n96 = call-poly <vilib>:"PID Lead-Lag.vi"() -> ()  [unwired: 8 in, 2 out]
              n97 = while {
                stop <- w113 stop-if-true
                # "Max Voltage"
                n98 = local read "Channel Array"() -> (w116:dbl[])
                n99 = call "OnDemand_VoltageOutput.vi"("Channel Array"=w116, "minimum voltage"=0.0, "maximum voltage"=5.067, "physical channels"="cDAQ9189-21D2231Mod6/ao0") -> ("error out"=→"error out":errorcluster)  [unwired: 7 in]
                n100 = global read "STOP_GLOBAL.vi" "ALL STOP"() -> (w113:bool)
              }
              n101 = while {
                stop <- w112 stop-if-true
                # "Max Voltage"
                n102 = call "OnDemand_VoltageOutput.vi"("Channel Array"="Array 2", "minimum voltage"=0.0, "maximum voltage"=10.0, "physical channels"="cDAQ9189-21D2231Mod6/ao1") -> ("error out"=→"error out 4":errorcluster)  [unwired: 7 in]
                n103 = global read "STOP_GLOBAL.vi" "ALL STOP"() -> (w112:bool)
              }
            }
            frame "Step Input" {
              # "Will wait 3 seconds to start, change in step every second"
              n104 = case shown="True" "PRESS TO START" {
                frame False {
                  # "Max Voltage"
                  n105 = call "OnDemand_VoltageOutput.vi"("Channel Array"=dbl[] [0.0], "minimum voltage"=0.0, "maximum voltage"=5.067, "physical channels"="cDAQ9189-21D2231Mod6/ao0") -> ()  [unwired: 7 in, 1 out]
                }
                frame True {
                  n106 = stacked-sequence {
                    seq-local: [_ _ _ _ _ w245 _ _ _] -> [_ _ _ _ _ _ w255 _ _]
                    seq-local: [_ _ _ _ _ _ w254 _ _] -> [_ _ _ _ _ _ _ w264 _]
                    seq-local: [w202 _ _ _ _ _ _ _ _] -> [_ w208 _ _ _ _ _ _ _]
                    seq-local: [_ w207 _ _ _ _ _ _ _] -> [_ _ _ w225 _ _ _ _ _]
                    seq-local: [_ _ _ w224 _ _ _ _ _] -> [_ _ _ _ w235 _ _ _ _]
                    seq-local: [_ _ _ _ w234 _ _ _ _] -> [_ _ _ _ _ w244 _ _ _]
                    frame #0 {
                      w202 = dbl[] [0.0]
                      # "Rest state for 3 sec"
                      # "Max Voltage"
                      n107 = call "OnDemand_VoltageOutput.vi"("Channel Array"=w202, "minimum voltage"=0.0, "maximum voltage"=5.067, "physical channels"="cDAQ9189-21D2231Mod6/ao0") -> ()  [unwired: 7 in, 1 out]
                      n108 = Wait (ms)(milliseconds to wait=u32 3000) -> ()  [unwired: 1 out]
                    }
                    frame #1 {
                      w209 = 6
                      n109 = for {
                        N: w209 -> [_]
                        shift-right: [w210] -> w207
                        shift-left: w208 -> [w217]
                        tunnel: w209 -> [w211]
                        # "Max Voltage"
                        n110 = Divide(x=5.067, y=w211) -> (x/y=w213:dbl)
                        n111 = Add(x=w217, y=w213) -> (x+y=w210:dbl[])
                        "Steps on Servo" <- w210
                        n112 = Wait (ms)(milliseconds to wait=u32 500) -> ()  [unwired: 1 out]
                        n113 = call "OnDemand_VoltageOutput.vi"("Channel Array"=w210, "minimum voltage"=0.0, "maximum voltage"=5.067, "physical channels"="cDAQ9189-21D2231Mod6/ao0") -> ()  [unwired: 7 in, 1 out]
                      }
                    }
                    frame #2 {
                      # "Max Voltage"
                      n114 = call "OnDemand_VoltageOutput.vi"("Channel Array"=dbl[] [5.067], "minimum voltage"=0.0, "maximum voltage"=5.067, "physical channels"="cDAQ9189-21D2231Mod6/ao0") -> ()  [unwired: 7 in, 1 out]
                      n115 = Wait (ms)(milliseconds to wait=u32 4000) -> ()  [unwired: 1 out]
                    }
                    frame #3 {
                      w226 = 6
                      n116 = for {
                        N: w226 -> [_]
                        shift-right: [w227] -> w224
                        shift-left: w225 -> [w233]
                        tunnel: w226 -> [_]
                        # "Max Voltage"
                        # "Until it reaches 2.067"
                        # "Reduce in steps of 0.5"
                        n117 = Subtract(x=w233, y=0.5) -> (x-y=w227:dbl[])
                        n118 = local write "Steps on Servo"(w227) -> ()
                        n119 = Wait (ms)(milliseconds to wait=u32 500) -> ()  [unwired: 1 out]
                        n120 = call "OnDemand_VoltageOutput.vi"("Channel Array"=w227, "minimum voltage"=0.0, "maximum voltage"=5.067, "physical channels"="cDAQ9189-21D2231Mod6/ao0") -> ()  [unwired: 7 in, 1 out]
                      }
                    }
                    frame #4 {
                      w236 = 6
                      n121 = for {
                        N: w236 -> [_]
                        shift-right: [w237] -> w234
                        shift-left: w235 -> [w243]
                        tunnel: w236 -> [_]
                        # "Max Voltage"
                        # "Until it reaches 2.067"
                        # "Increase in steps of 0.5"
                        n122 = Add(x=w243, y=0.5) -> (x+y=w237:dbl[])
                        n123 = local write "Steps on Servo"(w237) -> ()
                        n124 = Wait (ms)(milliseconds to wait=u32 500) -> ()  [unwired: 1 out]
                        n125 = call "OnDemand_VoltageOutput.vi"("Channel Array"=w237, "minimum voltage"=0.0, "maximum voltage"=5.067, "physical channels"="cDAQ9189-21D2231Mod6/ao0") -> ()  [unwired: 7 in, 1 out]
                      }
                    }
                    frame #5 {
                      w246 = 6
                      n126 = for {
                        N: w246 -> [_]
                        shift-right: [w247] -> w245
                        shift-left: w244 -> [w253]
                        tunnel: w246 -> [_]
                        # "Max Voltage"
                        # "Until it reaches 2.067"
                        # "Reduce in steps of 0.5"
                        n127 = Subtract(x=w253, y=0.5) -> (x-y=w247:dbl[])
                        n128 = local write "Steps on Servo"(w247) -> ()
                        n129 = Wait (ms)(milliseconds to wait=u32 500) -> ()  [unwired: 1 out]
                        n130 = call "OnDemand_VoltageOutput.vi"("Channel Array"=w247, "minimum voltage"=0.0, "maximum voltage"=5.067, "physical channels"="cDAQ9189-21D2231Mod6/ao0") -> ()  [unwired: 7 in, 1 out]
                      }
                    }
                    frame #6 {
                      n131 = for {
                        N: 6 -> [_]
                        shift-right: [w257] -> w254
                        shift-left: w255 -> [w263]
                        # "Max Voltage"
                        # "Until it reaches 2.067"
                        # "Increase in steps of 0.5"
                        n132 = Add(x=w263, y=0.5) -> (x+y=w257:dbl[])
                        n133 = local write "Steps on Servo"(w257) -> ()
                        n134 = Wait (ms)(milliseconds to wait=u32 500) -> ()  [unwired: 1 out]
                        n135 = call "OnDemand_VoltageOutput.vi"("Channel Array"=w257, "minimum voltage"=0.0, "maximum voltage"=5.067, "physical channels"="cDAQ9189-21D2231Mod6/ao0") -> ()  [unwired: 7 in, 1 out]
                      }
                    }
                    frame #7 {
                      w265 = 6
                      n136 = for {
                        N: w265 -> [_]
                        shift-right: [w266] -> _
                        shift-left: w264 -> [w272]
                        tunnel: w265 -> [_]
                        # "Max Voltage"
                        # "Until it reaches 2.067"
                        # "reduce in steps of 0.5"
                        n137 = Subtract(x=w272, y=0.5) -> (x-y=w266:dbl[])
                        n138 = local write "Steps on Servo"(w266) -> ()
                        n139 = Wait (ms)(milliseconds to wait=u32 500) -> ()  [unwired: 1 out]
                        n140 = call "OnDemand_VoltageOutput.vi"("Channel Array"=w266, "minimum voltage"=0.0, "maximum voltage"=5.067, "physical channels"="cDAQ9189-21D2231Mod6/ao0") -> ()  [unwired: 7 in, 1 out]
                      }
                    }
                    frame #8 {
                      w273 = dbl[] [0.0]
                      # "Reset to 0"
                      # "Max Voltage"
                      n141 = call "OnDemand_VoltageOutput.vi"("Channel Array"=w273, "minimum voltage"=0.0, "maximum voltage"=5.0, "physical channels"="cDAQ9189-21D2231Mod6/ao0") -> ()  [unwired: 7 in, 1 out]
                      n142 = local write "Steps on Servo"(w273) -> ()
                    }
                  }
                  n143 = while {
                    stop <- w201 stop-if-true
                    n144 = call "Elapsed Time2"() -> ("Elapsed Time (s)"=w199:dbl)  [unwired: 12 in, 7 out]
                    "Elapsed Time (s) 2" <- w199
                    n145 = global read "STOP_GLOBAL.vi" "ALL STOP"() -> (w201:bool)
                    n146 = Greater?(x=w199, y=3.0 ("x")) -> (0:→"HAS 3 SECONDS PASSED?":bool)
                  }
                }
              }
            }
            frame "Do nothing" {
            }
          }
          n147 = call <vilib>:"High Resolution Relative Seconds.vi"() -> ("relative seconds"=w51:dbl)
          n148 = while {
            tunnel: "Types of Testing" -> [w303]
            tunnel: [w340] -> w65 mode=indexing
            shift-right: [w332] -> w69
            shift-left: w48 -> [w335]
            shift-right: [w308] -> w70
            shift-left: w49 -> [w334]
            tunnel: [w317] -> w66 mode=indexing
            tunnel: [w315] -> w62 mode=indexing
            tunnel: [w314] -> w67 mode=indexing
            tunnel: [w313] -> w68 mode=indexing
            tunnel: [w309] -> w53 mode=indexing
            tunnel: [w292] -> w61 mode=indexing
            tunnel: [w316] -> w60 mode=indexing
            tunnel: w51 -> [w295]
            tunnel: w50 -> [w291]
            tunnel: w46 -> [w290]
            i -> [w341]
            stop <- w278 stop-if-true
            w328 = 110.0 ("x")
            w338 = 1.0  # timeout (s)
            # "Add SetPoint History\nAdd Gain history to data"
            # "First Test:\n2.1\n70\n3.566\nSecond:\n2.1\n80\n3.566\nThird:\n3.1\n60\n3.566\nFourth:\n10.1\n70\n3.566"
            # "Supply\nSecond Transducer\nFlow\nTemp\nOutput Voltage"
            # "4 NI 9219 Channels"
            # "Combined Loop cDAQ"
            n149 = call <vilib>:"High Resolution Relative Seconds.vi"() -> ("relative seconds"=w296:dbl)
            n150 = Subtract(x=w296, y=w295) -> (x-y=w293:dbl)
            n151 = Subtract(x=w293, y=0.0) -> (x-y=w292:dbl)
            "Entire Runtime" <- w292
            n152 = local read "Actual Clock Rate"() -> (w298:dbl)
            n153 = call-poly <vilib>:"DAQmx Read.vi"("task/channels in"=w334, "number of samples per channel"=w291, "timeout"=w338, "error in"=w335) -> ("task out"=w308:refnum<k21>, "data"=w336:waveform(dbl)[], "error out"=w332:errorcluster)  [unwired: 9 in]
            n154 = local read "SP"() -> (w280:dbl)
            n155 = global read "STOP_GLOBAL.vi" "ALL STOP"() -> (w337:bool)
            n156 = Split Signals(w336) -> (w288:dynamicdata, w287:dynamicdata, w284:dynamicdata, w331:dynamicdata, w282:dynamicdata, w330:dynamicdata, w283:dynamicdata)  [unwired: 15 in, 8 out]
            n157 = Unbundle By Name(w332) -> ("status"=w339:bool)
            n158 = Divide(x=1.0, y=w298) -> (x/y=w297:dbl)
            n159 = Greater?(x=w280, y=0.0) -> (0:w279:bool)
            n160 = case shown="True" w279 {
              tunnel: [FALSE w343] -> w277
              frame False {
              }
              frame True {
                n161 = call "Elapsed Time"() -> ("Elapsed Time (s)"=w344:dbl)  [unwired: 12 in, 7 out]
                "Elapsed Time (s)" <- w344
                n162 = local read "RunTime"() -> (w345:dbl)
                n163 = Greater?(x=w344, y=w345) -> (0:w343:bool)
              }
            }
            "Stop" <- w277
            n164 = Multiply(x=1000.0, y=w297) -> (x*y=w289:dbl)
            n165 = Or(x=w339, y=w337) -> (x .or. y?=w278:bool)
            n166 = Wait Until Next ms Multiple(millisecond multiple=w289) -> ()  [unwired: 1 out]
            n167 = Merge Signals(w284, w331, w282, w330, w283, w288, w287) -> (w329:dynamicdata)
            n168 = call "Filter3"("Signal"=w329) -> ("Filtered Signal"=w326:dynamicdata)  [unwired: 9 in, 1 out]
            n169 = Split Signals(w326) -> (w307:dynamicdata, w306:dynamicdata, w305:dynamicdata, w304:dynamicdata, w301:dynamicdata, w286:dynamicdata, w285:dynamicdata)  [unwired: 7 in]
            n170 = local write "Temperature"(w285) -> ()
            n171 = Merge Signals(w307, w306, w304, w285, w301) -> (w333:dynamicdata)
            n172 = local write "Voltage Output"(w301) -> ()
            n173 = Merge Signals(w307, w306, w305, w304, w286, w285, w301) -> (w302:dynamicdata)
            n174 = Multiply(x=w328, y=w307) -> (x*y=w325:dynamicdata)
            n175 = Multiply(x=w328, y=w306) -> (x*y=w322:dynamicdata)
            n176 = Multiply(x=w328, y=w305) -> (x*y=w321:dynamicdata)
            n177 = Multiply(x=200.0, y=w304) -> (x*y=w319:dynamicdata)
            n178 = case shown="\"Test Firing\", Default" w303 {
              tunnel: w333 -> [_ w371]
              tunnel: w302 -> [w354 _]
              tunnel: w290 -> [w346 w362]
              frame "Test Firing", Default {
                n179 = Build Array("Supply Pressure", "Second Pressure Transducer", "Chamber Pressure", "Volumetric Flow", "Thrust", "Temperature", "Voltage Out" ("element")) -> (w352:string[])
                n180 = call "RenameDynamicSignals.vi"("New Signal Names"=w352, "Dynamic Data In"=w354) -> ("error out"=w350:errorcluster, "Dynamic Data Out"=w351:dynamicdata)  [unwired: 2 in]
                n181 = call "Write To Measurement File3"("Signals"=w351, "Enable"="Collect Data?", "error in (no error)"=w350, "Filename"=w346) -> ("Filename Out"=→"Filename Out":path, "Saving Data"=→"Saving Data":bool, "error out"=→"error out 3":errorcluster)  [unwired: 13 in]
              }
              frame "Cold Flow Rig" {
                n182 = Build Array("Supply Pressure", "Second Pressure Transducer", "Volumetric Flow", "Temperature", "Voltage Out" ("element")) -> (w365:string[])
                n183 = call "RenameDynamicSignals.vi"("New Signal Names"=w365, "Dynamic Data In"=w371) -> ("error out"=w363:errorcluster, "Dynamic Data Out"=w364:dynamicdata)  [unwired: 2 in]
                n184 = call "Write To Measurement File4"("Signals"=w364, "Enable"="Collect Data? 2", "error in (no error)"=w363, "Filename"=w362) -> ("Filename Out"=→"Filename Out":path, "Saving Data"=→"Saving Data":bool)  [unwired: 13 in, 1 out]
              }
            }
            n185 = local write "Supply Pressure PSI"(w325) -> ()
            n186 = local write "Chamber Pressure"(w321) -> ()
            n187 = local write "Second Pressure Transducer"(w322) -> ()
            n188 = local write "Mass Flow L/min"(w319) -> ()
            n189 = local write "Thrust lb"(w286) -> ()
            n190 = call "Convert from Dynamic Data11"("Dynamic Data Type"=w322) -> ("Array"=w323:dbl[])  [unwired: 3 in]
            n191 = call "Convert from Dynamic Data8"("Dynamic Data Type"=w325) -> ("Array"=w324:dbl[])  [unwired: 3 in]
            n192 = call "Convert from Dynamic Data12"("Dynamic Data Type"=w321) -> ("Array"=w320:dbl[])  [unwired: 3 in]
            n193 = call "Convert from Dynamic Data13"("Dynamic Data Type"=w319) -> ("Array"=w318:dbl[])  [unwired: 3 in]
            n194 = call-poly <vilib>:"Mean.vi"("X"=w324) -> ("mean"=w317:dbl)  [unwired: 1 out]
            n195 = call-poly <vilib>:"Mean.vi"("X"=w323) -> ("mean"=w316:dbl)  [unwired: 1 out]
            n196 = call-poly <vilib>:"Mean.vi"("X"=w320) -> ("mean"=w315:dbl)  [unwired: 1 out]
            n197 = call-poly <vilib>:"Mean.vi"("X"=w318) -> ("mean"=w314:dbl)  [unwired: 1 out]
            n198 = call "Convert from Dynamic Data3"("Dynamic Data Type"=w285) -> ("Array"=w311:dbl[])  [unwired: 3 in]
            n199 = call "Convert from Dynamic Data4"("Dynamic Data Type"=w301) -> ("Array"=w310:dbl[])  [unwired: 3 in]
            n200 = call "Convert from Dynamic Data"("Dynamic Data Type"=w286) -> ("Array"=w312:dbl[])  [unwired: 3 in]
            n201 = call-poly <vilib>:"Mean.vi"("X"=w310) -> ("mean"=w309:dbl)  [unwired: 1 out]
            n202 = call-poly <vilib>:"Mean.vi"("X"=w312) -> ("mean"=w340:dbl)  [unwired: 1 out]
            n203 = call-poly <vilib>:"Mean.vi"("X"=w311) -> ("mean"=w313:dbl)  [unwired: 1 out]
            "Numeric 2" <- w341
          }
          "Array" <- w61
          n204 = call <vilib>:"DAQmx Clear Task.vi"("task in"=w70, "error in"=w69) -> ("error out"=→"error out 2":errorcluster)  [unwired: 13 in]
          n205 = Bundle(w61, w60) -> (w59:cluster{dbl[], dbl[]})  [unwired: 1 in]
          "Second Pressure Transducer" <- w59
          n206 = Bundle(w61, w62) -> (w58:cluster{dbl[], dbl[]})  [unwired: 1 in]
          "Chamber Pressure" <- w58
          n207 = Bundle(w61, w66) -> (w64:cluster{dbl[], dbl[]})  [unwired: 1 in]
          "Supply Pressure" <- w64
          n208 = Bundle(w61, w67) -> (w57:cluster{dbl[], dbl[]})  [unwired: 1 in]
          "MassFlow" <- w57
          n209 = Bundle(w61, w65) -> (w56:cluster{dbl[], dbl[]})  [unwired: 1 in]
          "Thrust" <- w56
          n210 = Bundle(w61, w68) -> (w55:cluster{dbl[], dbl[]})  [unwired: 1 in]
          "Temperature" <- w55
          n211 = Bundle(w61, w53) -> (→"Servo Voltage Output":cluster{dbl[], dbl[]})  [unwired: 1 in]
          n212 = Build Array(w64, w59, w58, w57, w56, w55) -> (→"All Channel Graph":cluster{dbl[], dbl[]}[])
        }
      }
    }
  }
